vi "_macro_Choreo_Command.vi"() -> ()   [LabVIEW 2019, in "ChoreoLib.lvlib"]
uses:
  ChoreoLib.lvlib
  <vilib>/Rock Robotics/WPI/ThirdParty/JAS_Junk/TrajLib/TypeDef/POSE2D.ctl
  <vilib>/Rock Robotics/WPI/ThirdParty/JAS_Junk/TrajLib/TypeDef/TRANSLATION2D.ctl
  <vilib>/Rock Robotics/WPI/ThirdParty/JAS_Junk/TrajLib/TypeDef/ROTATION2D.ctl
  TypeDef/ChoreoTrajectory.ctl
  TypeDef/ChoreoTrajectoryState.ctl
  <vilib>/Rock Robotics/WPI/ThirdParty/JAS_Junk/TrajLib/VI/numCmd_Send_Generic.vi
  <vilib>/Rock Robotics/WPI/ThirdParty/JAS_Junk/TrajLib/VI/numCmd_ObtainQueue_Generic.vi
  <vilib>/Rock Robotics/WPI/ThirdParty/JAS_Junk/TrajLib/Trajectory_Library.lvlib
panel:
  in  "Initialize":bool
  in  "ChoreoTrajectory":T1
  in  "Current Position":T3={"TRANSLATION"={"X"=0.0, "Y"=0.0}, "ROTATION"={"VALUE"=0.0, "COS"=1.0, "SIN"=0.0}} {"ROTATION"."SIN" format="%13.4f"; "ROTATION"."COS" format="%13.4f"; "ROTATION"."VALUE" format="%13.4f"; "TRANSLATION"."Y" format="%14.3f"; "TRANSLATION"."X" format="%14.3f"}
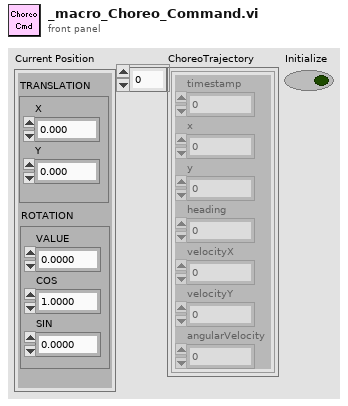
[diagram p1: front panel]
types:
  T1 = typedef "ChoreoLib.lvlib/ChoreoTrajectory.ctl" = T2[]
  T2 = typedef "ChoreoLib.lvlib/ChoreoTrajectoryState.ctl" = cluster{"timestamp":dbl, "x":dbl, "y":dbl, "heading":dbl, "velocityX":dbl, "velocityY":dbl, "angularVelocity":dbl}
  T3 = typedef "Trajectory_Library.lvlib/POSE2D.ctl" = cluster{"TRANSLATION":T4, "ROTATION":T5}
  T4 = typedef "Trajectory_Library.lvlib/TRANSLATION2D.ctl" = cluster{"X":dbl, "Y":dbl}
  T5 = typedef "Trajectory_Library.lvlib/ROTATION2D.ctl" = cluster{"VALUE":dbl, "COS":dbl, "SIN":dbl}
  T6 = typedef "Trajectory_Library.lvlib/PID_ADV_LIMITS.ctl" = cluster{"MaxInput":dbl, "MinInput":dbl, "Continuous":bool, "MaxOutput":dbl, "MinOutput":dbl}
  T7 = typedef "Trajectory_Library.lvlib/PID_ADV_TUNING.ctl" = cluster{"Kf":dbl, "Kp":dbl, "Ki":dbl, "Kd":dbl, "MaximumIntegral":dbl, "MinimumIntegral":dbl, "Filter Derivative":bool}
  T8 = typedef "ChoreoLib.lvlib/ChoreoSwerveControlConfig.ctl" = cluster{"X_Adv PID Tuning":T7, "X_Adv PID Limits":T6, "Y_Adv PID Tuning":T7, "Y_Adv PID Limits":T6, "Rot_Adv PID Tuning":T7, "Rot_Adv PID Limits":T6, "X Y Pos Tolerance M":dbl, "Rot Tolerance Deg":dbl, "X Y Vel Tolerance M/S":dbl, "Rot Vel Tolerance Deg/S":dbl}
  T9 = typedef "Trajectory_Library.lvlib/CHASSIS_SPEEDS.ctl" = cluster{"vX":dbl, "vY":dbl, "vOmega":dbl}
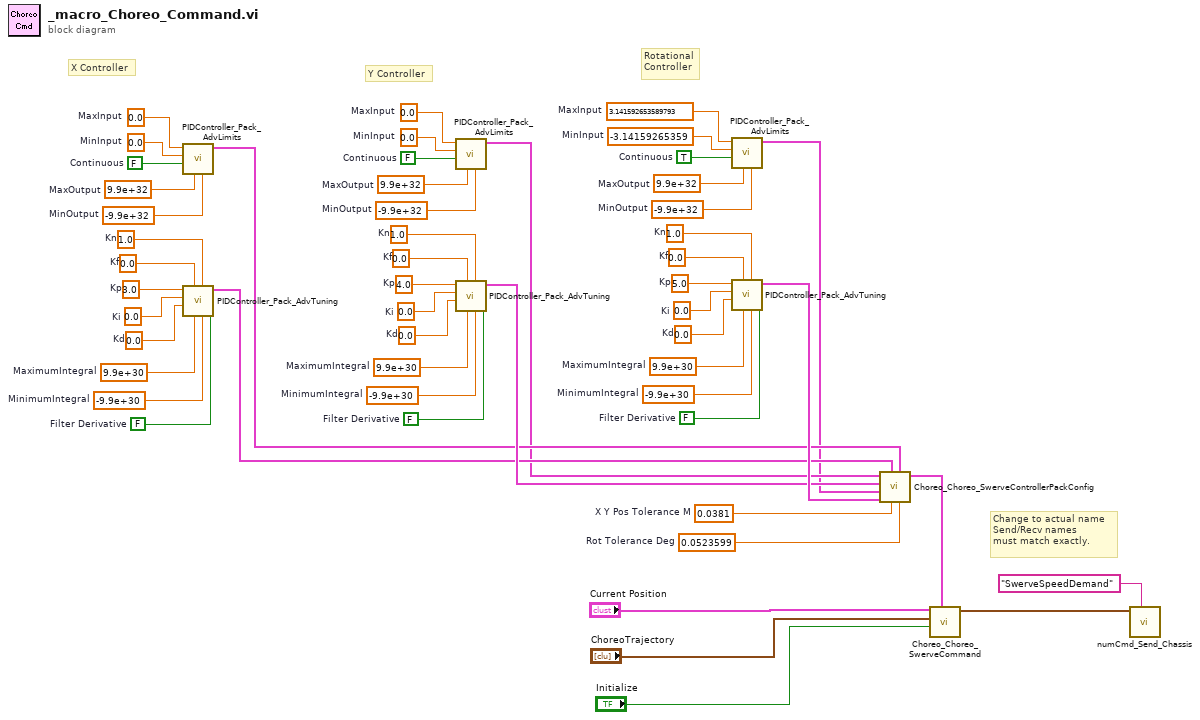
[diagram p0: block diagram]
diagram:
  w1 = 0.0523599  # Rot Tolerance Deg
  w2 = 0.0381  # X Y Pos Tolerance M
  w26 = 1.0  # Kn
  w25 = 5.0  # Kp
  w24 = 0.0  # Ki
  w23 = 0.0  # Kd
  w22 = 0.0  # Kf
  w21 = 9.9e+30  # MaximumIntegral
  w20 = -9.9e+30  # MinimumIntegral
  w19 = FALSE  # Filter Derivative
  w17 = -3.14159265359  # MinInput
  w16 = TRUE  # Continuous
  w15 = 9.9e+32  # MaxOutput
  w18 = -9.9e+32  # MinOutput
  w14 = 3.141592653589793  # MaxInput
  w39 = 1.0  # Kn
  w38 = 4.0  # Kp
  w37 = 0.0  # Ki
  w36 = 0.0  # Kd
  w35 = 0.0  # Kf
  w34 = 9.9e+30  # MaximumIntegral
  w33 = -9.9e+30  # MinimumIntegral
  w32 = FALSE  # Filter Derivative
  w30 = 0.0  # MinInput
  w29 = FALSE  # Continuous
  w28 = 9.9e+32  # MaxOutput
  w31 = -9.9e+32  # MinOutput
  w27 = 0.0  # MaxInput
  w52 = 1.0  # Kn
  w51 = 3.0  # Kp
  w50 = 0.0  # Ki
  w49 = 0.0  # Kd
  w48 = 0.0  # Kf
  w47 = 9.9e+30  # MaximumIntegral
  w46 = -9.9e+30  # MinimumIntegral
  w45 = FALSE  # Filter Derivative
  w43 = 0.0  # MinInput
  w42 = FALSE  # Continuous
  w41 = 9.9e+32  # MaxOutput
  w44 = -9.9e+32  # MinOutput
  w40 = 0.0  # MaxInput
  # "Change to actual name\nSend/Recv names\nmust match exactly."
  # "Rotational\nController"
  # "Y Controller"
  # "X Controller"
  n1 = call <vilib>:"PIDController_Pack_AdvLimits.vi"("MinOutput"=w44, "MaxOutput"=w41, "Continuous"=w42, "MinInput"=w43, "MaxInput"=w40) -> ("Adv PID Limits"=w5:T6)  [unwired: 6 in]
  n2 = call <vilib>:"PIDController_Pack_AdvTuning.vi"("Filter Derivative"=w45, "MinimumIntegral"=w46, "Kn"=w52, "MaximumIntegral"=w47, "Kf"=w48, "Kd"=w49, "Ki"=w50, "Kp"=w51) -> ("Adv PID Tuning"=w11:T7)  [unwired: 3 in]
  n3 = call <vilib>:"PIDController_Pack_AdvLimits.vi"("MinOutput"=w31, "MaxOutput"=w28, "Continuous"=w29, "MinInput"=w30, "MaxInput"=w27) -> ("Adv PID Limits"=w4:T6)  [unwired: 6 in]
  n4 = call <vilib>:"PIDController_Pack_AdvTuning.vi"("Filter Derivative"=w32, "MinimumIntegral"=w33, "Kn"=w39, "MaximumIntegral"=w34, "Kf"=w35, "Kd"=w36, "Ki"=w37, "Kp"=w38) -> ("Adv PID Tuning"=w12:T7)  [unwired: 3 in]
  n5 = call <vilib>:"PIDController_Pack_AdvLimits.vi"("MinOutput"=w18, "MaxOutput"=w15, "Continuous"=w16, "MinInput"=w17, "MaxInput"=w14) -> ("Adv PID Limits"=w3:T6)  [unwired: 6 in]
  n6 = call <vilib>:"PIDController_Pack_AdvTuning.vi"("Filter Derivative"=w19, "MinimumIntegral"=w20, "Kn"=w26, "MaximumIntegral"=w21, "Kf"=w22, "Kd"=w23, "Ki"=w24, "Kp"=w25) -> ("Adv PID Tuning"=w13:T7)  [unwired: 3 in]
  n7 = call "Choreo_Choreo_SwerveControllerPackConfig.vi"("Rot Tolerance Deg"=w1, "X_Adv PID Limits"=w5, "X Y Pos Tolerance M"=w2, "X_Adv PID Tuning"=w11, "Rot_Adv PID Tuning"=w13, "Rot_Adv PID Limits"=w3, "Y_Adv PID Tuning"=w12, "Y_Adv PID Limits"=w4) -> ("ChoreoSwerveControlConfig"=w53:T8)  [unwired: 3 in]
  n8 = call "Choreo_Choreo_SwerveCommand.vi"("ChoreoSwerveControlConfig"=w53, "Initialize"="Initialize", "ChoreoTrajectory"="ChoreoTrajectory", "Current Position"="Current Position") -> ("Chassis Speed Dmd"=w6:T9)  [unwired: 4 in, 3 out]
  n9 = call <vilib>:"numCmd_Send_Chassis.vi"("Command Name"="SwerveSpeedDemand", "Chassis Speeds"=w6) -> ()  [unwired: 9 in, 1 out]
